vi "LvDatatypeToImageType_EXT.vi"(9 "error in":errorcluster, 11 "Numeric":ext) -> (1 "error out":errorcluster, 2 "Image Type":T1, 3 "Numeric out":ext)   [LabVIEW 2020, in "OpenLvVision_OpenCv.lvlib"]
doc: "converts 2d array to image format"
uses:
  OpenLvVision_OpenCv.lvlib
  <vilib>/OpenLvVision/OpenLvVision_Image/Management/TypeDef/OLV ImageType.ctl
  <vilib>/Utility/error.llb/Error Cluster From Error Code.vi
  <vilib>/ErrorRing/Error Ring.xnode
  <vilib>/OpenLvVision/OpenLvVision_Image/Management/OLV Management.lvlib
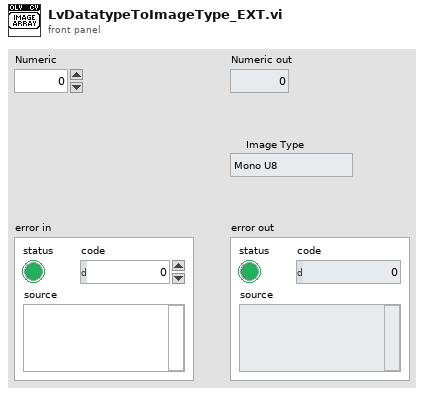
[diagram p1: front panel]
types:
  T1 = typedef "OLV OpenLvVision_Image.lvlib/OLV Management.lvlib/OLV ImageType.ctl" = enum16{"Mono U8", "Mono U16", "Mono I16", "Mono SGL", "Color U32", "Color U64", "Complex CSG"}
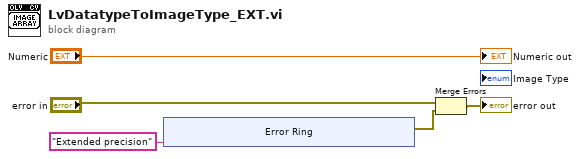
[diagram p0: block diagram]
diagram:
  n1 = xnode "Error Ring"("parameter 0"="Extended precision") -> ("error out"=w4:errorcluster)
  n2 = Merge Errors("error in", w4) -> (→"error out":errorcluster)
  "Numeric out" <- "Numeric"
